vi "WT210 Basic Reset.vi"(8 "error in (no error)":errorcluster, 9 "V Range (6: 600V)":u16(ring)=4 items=["Auto", "15V", "30V", "60V", "150V", "300V", "600V"], 10 "A Range (12: 20A)":u16(ring)=10 items=["Auto", "5mA", "10mA", "20mA", "50mA", "100mA", "200mA", "0.5A", "1A", "2A", "5A", "10A", "20A", "50mV", "100mV", "200mV", "2.5V", "5V", "10V"], 11 "VISA Refnum in":refnum<visa-resource-name>) -> (0 "error out":errorcluster, 1 "Sample Rate (1: 0.25s)":u16(ring)=1 items=["0.1s", "0.25s", "0.5s", "1s", "2s", "5s"], 2 "Instrument ID":string, 3 "VISA Refnum out":refnum<visa-resource-name>)   [LabVIEW 2019]
uses:
  Yokogawa WT200 Series.lvlib
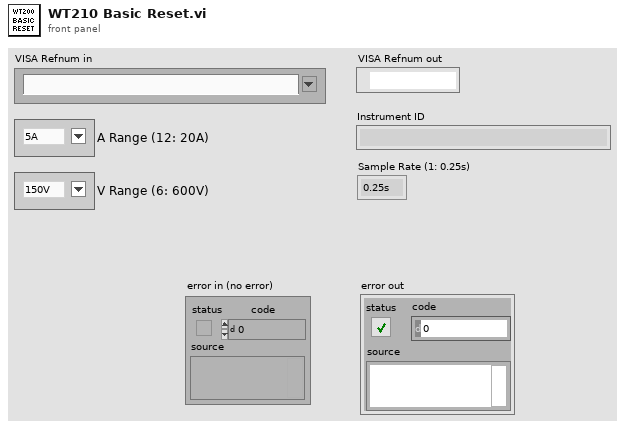
[diagram p1: front panel]
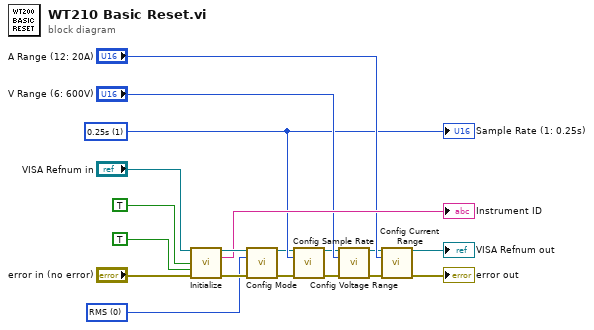
[diagram p0: block diagram]
diagram:
  w11 = u16 1 items=["0.1s", "0.25s", "0.5s", "1s", "2s", "5s"] ("Sample Rate (1: 0.25s)")
  w8 = u16 0 items=["RMS", "V-MEAN", "DC"] ("Mode (0: RMS)")
  n1 = call "Initialize.vi"("VISA resource name"="VISA Refnum in", "ID Query (T: Check)"=TRUE, "Reset (T: Reset)"=TRUE, "error in (no error)"="error in (no error)") -> ("VISA resource name out"=w18:refnum<visa-resource-name>, "Instrument ID"=→"Instrument ID":string, "error out"=w17:errorcluster)  [unwired: 9 in]
  n2 = call "Config Mode.vi"("VISA resource name"=w18, "Mode (0: RMS)"=w8, "error in (no error)"=w17) -> ("VISA resource name out"=w10:refnum<visa-resource-name>, "error out"=w9:errorcluster)  [unwired: 11 in]
  n3 = call "Config Sample Rate.vi"("VISA resource name"=w10, "Sample Rate (1: 0.25s)"=w11, "error in (no error)"=w9) -> ("VISA resource name out"=w4:refnum<visa-resource-name>, "error out"=w2:errorcluster)  [unwired: 11 in]
  n4 = call "Config Voltage Range.vi"("VISA resource name"=w4, "V Range (6: 600V)"="V Range (6: 600V)", "error in (no error)"=w2) -> ("VISA resource name out"=w5:refnum<visa-resource-name>, "error out"=w3:errorcluster)  [unwired: 11 in]
  n5 = call "Config Current Range.vi"("VISA resource name"=w5, "A Range (12: 20A)"="A Range (12: 20A)", "error in (no error)"=w3) -> ("VISA resource name out"=→"VISA Refnum out":refnum<visa-resource-name>, "error out"=→"error out":errorcluster)  [unwired: 11 in]
  "Sample Rate (1: 0.25s)" <- w11
